vi "Options GFV.vi"(2 "Anything":variant, 5 "error in (no error)":errorcluster, 6 "Action(Get Settings)":T20=enum."Get Settings", 7 "Setting ID":T19=enum."P 2") -> (14 "Update index":i32, 16 "Options":T1={"P 1 (App)"={"Result files"=path "", "PCP Interface"="", "Tractor/Stroker Interface"="", "Tractor Interface"="", "Modem Status Interface"="", "Audible Alarm"=FALSE, "Force alarm on Technical"=FALSE, "Force alarm on HH"=FALSE, "Force alarm on LL"=FALSE, "Force alarm on H"=FALSE, "Force alarm on L"=FALSE}, "P 2"={"Solenoid & Relay latching time"=0, "Tractor relay 1"=0.3, "Tractor relay 2"=0.2, "Tractor Solenoid limit"=0.2}, "P 3"={"Min resistance"=0.0, "Max resistance"=0.0, "Head voltage range"=enum."0 - 350V", "Max voltage jump"=40.0, "Maximum resistance change"=40.0, "Start Telemetry Voltage"=35.0, "Start Telemetry Timeout"=160.0, "Start Motor Voltage"=1.0, "Stop Motor Voltage"=1.0, "Pass Mode Warning Voltage"=1.0, "Relay Switch Voltage"=160.0, "Relay Status Loss Voltage"=0.0, "Samples to average"=1, "PSU type DO NOT USE"=enum."Magna 8.3A", "Magna OVP"=1.0, "Magna Current Limit"=160.0}, "P 4"={"Solenoid & Relay latching time"=40, "Stroker relay 1"=1.0, "Stroker Relay 2"=40.0, "Stroker Solenoid limit"=0.0, "Force det."=enum."Stroke in = node 1", "Stroke force lim."=0.0, "Anchor Enabled Pressure"=0.05, "Tacometer puls"=0.3, "Default anchor behavior"=enum."Do nothing", "Default stroker behavior"=enum."Do nothing", "Default stroker force limit (tonne)"=0.0, "Slips Size"=enum."338 MRS"}, "P 5"={"Solenoid & Relay latching time"=0, "Driller relay 1"=0.3, "Driller Relay 2"=0.2, "Driller  Solenoid limit"=0.2}, "P 6 (Err)"={"Error and event files"=path ""}, "P 7 (Expert)"={"Show Debug"=FALSE, "Log debug messages"=FALSE, "Additional debug messages"=FALSE, "Start Beagle with Simulator data"=FALSE, "Workshop mode"=FALSE, "Modem baud"=38400, "enumCANCOM"=FALSE, "Modem sim"={"Modem dealay sim"=FALSE, "Sim baud Tx"=1200, "Bit Error fraction Tx"=0.0, "Sim baud Rx"=1200, "Bit Error fraction Rx"=0.0}, "Telemetry Timeout Disable"=20, "Buffer size"=20, "Upd regular data"=FALSE, "Cable comp"={"VMOD1 Voltage(V)"=1.0, "VMOD2 Voltage(V)"=8.0}}, "P 8 (Depth)"={"Winch Spool Circumference"=100.0, "Winch Pulses per Revolution"=160.0, "Current Depth"=100.0}, "C 1"={"Depth Updated"=FALSE, "Depth Offset"=0.0}, "C 2"={"Placeholder"=FALSE}} {"P 8 (Depth)"."Current Depth" format="%#.7f"; "P 8 (Depth)"."Winch Pulses per Revolution" min=1.0 max=100000.0 step=1.0 format="%#.0f"; "P 8 (Depth)"."Winch Spool Circumference" min=0.0 max=200.0 format="%#.7f"; "C 1"."Depth Offset" format="%#.7f"; "P 2"."Tractor Solenoid limit" format="%.2f"; "P 2"."Tractor relay 2" format="%.2f"; "P 2"."Tractor relay 1" format="%.2f"; "P 3"."Relay Status Loss Voltage" min=0.0 max=500.0 format="%#.0f"; "P 3"."Relay Switch Voltage" min=5.0 max=500.0 format="%#.0f"; "P 3"."Magna Current Limit" min=0.0 max=20.0 format="%.1f"; "P 3"."Magna OVP" min=0.0 max=1500.0 format="%#.0f"; "P 3"."Pass Mode Warning Voltage" min=5.0 max=500.0 format="%#.0f"; "P 3"."Stop Motor Voltage" min=5.0 max=500.0 format="%#.0f"; "P 3"."Start Telemetry Timeout" min=0.0 max=500.0 format="%#.0f"; "P 3"."Samples to average" min=1 max=10; "P 3"."Start Motor Voltage" min=5.0 max=500.0 format="%#.0f"; "P 3"."Start Telemetry Voltage" min=5.0 max=500.0 format="%#.0f"; "P 3"."Maximum resistance change" min=1.0 max=100.0 format="%#.0f"; "P 3"."Max voltage jump" min=5.0 max=500.0 format="%#.0f"; "P 3"."Max resistance" min=30.0 max=500.0 format="%#.0f"; "P 3"."Min resistance" min=0.0 max=500.0 format="%#.0f"; "P 4"."Default stroker force limit (tonne)" format="%.2f"; "P 4"."Stroker Relay 2" format="%.2f"; "P 4"."Stroker relay 1" format="%.2f"; "P 4"."Tacometer puls" format="%.2f"; "P 4"."Anchor Enabled Pressure" format="%.2f"; "P 4"."Stroke force lim." format="%.2f"; "P 4"."Stroker Solenoid limit" format="%.2f"; "P 5"."Driller  Solenoid limit" format="%.2f"; "P 5"."Driller Relay 2" format="%.2f"; "P 5"."Driller relay 1" format="%.2f"; "P 7 (Expert)"."Cable comp"."VMOD2 Voltage(V)" format="%.1f"; "P 7 (Expert)"."Cable comp"."VMOD1 Voltage(V)" format="%.1f"; "P 7 (Expert)"."Telemetry Timeout Disable" min=2 max=20 step=2; "P 7 (Expert)"."Modem baud" items=["38400 (Normal use)"=38400, "9600 (Development)"=9600]; "P 7 (Expert)"."Modem sim"."Bit Error fraction Rx" format="%.9f"; "P 7 (Expert)"."Modem sim"."Sim baud Rx" items=["9600"=9600, "4800"=4800, "2400"=2400, "1200"=1200, "1000"=1000, "800"=800, "600"=600, "400"=400, "200"=200]; "P 7 (Expert)"."Modem sim"."Bit Error fraction Tx" format="%.9f"; "P 7 (Expert)"."Modem sim"."Sim baud Tx" items=["9600"=9600, "4800"=4800, "2400"=2400, "1200"=1200, "1000"=1000, "800"=800, "600"=600, "400"=400, "200"=200]; "P 7 (Expert)"."Buffer size" min=86400 max=1209600}, 19 "error out":errorcluster)   [LabVIEW 2011]
uses:
  Action GFV Settings.ctl
  Options PageID.ctl
  Options  All pages and custom.ctl
  Options Page 1 (App).ctl
  Options Page 2.ctl
  Options Page 3.ctl
  PCP interface/PCP type List.ctl
  PCP interface/PSU Type.ctl
  Options Page 4.ctl
  Tool/Stroke force selector.ctl
  Tool/Default anchor behavior.ctl
  Tool/Default stroker behavior.ctl
  GUI/Controls/Slips Type Radio.ctl
  Options Page 5.ctl
  Options Page 6 (Err).ctl
  Options Page 7 (Expert).ctl
  GUI/Options/Modem simulation setup.ctl
  Options Page 8 (Depth).ctl
  Options Custom 1.ctl
  Options Custom 2.ctl
  <vilib>/Utility/sysdir.llb/System Directory Type.ctl
  <vilib>/Utility/VariantDataType/GetNumericInfo.vi
  emi Lib/Basic/0 - General/App/Version/Private/_emi_Version Holder.vi
  emi Lib/System 01/0 - General/Debug/Private/_emi_GFV Debug Disp.vi
  emi Lib/System 01/0 - General/Debug/Private/_emi_GFV Debug Log.vi
  emi Lib/System 01/0 - General/Debug/Private/_emi_GFV Debug Aditional.vi
  <vilib>/Utility/libraryn.llb/Check if File or Folder Exists.vi
panel:
  # "m"
  # "Pulses"
  # "Not meant to be directly displayed"
  # "Not meant to be directly displayed"
  # "ms"
  # "When both relays are used in \nthe same operation, the lowest\nlimit is used for both."
  # "A"
  # "A"
  # "A"
  # "Ohm"
  # "Ohm"
  # "V"
  # "Ohm"
  # "V"
  # "s"
  # "V"
  # "V"
  # "V"
  # "V"
  # "V"
  # "ms"
  # "When both relays are used in \nthe same operation, the lowest\nlimit is used for both."
  # "A"
  # "A"
  # "A"
  # "Bar"
  # "ms"
  # "When both relays are used in \nthe same operation, the lowest\nlimit is used for both."
  # "A"
  # "A"
  # "A"
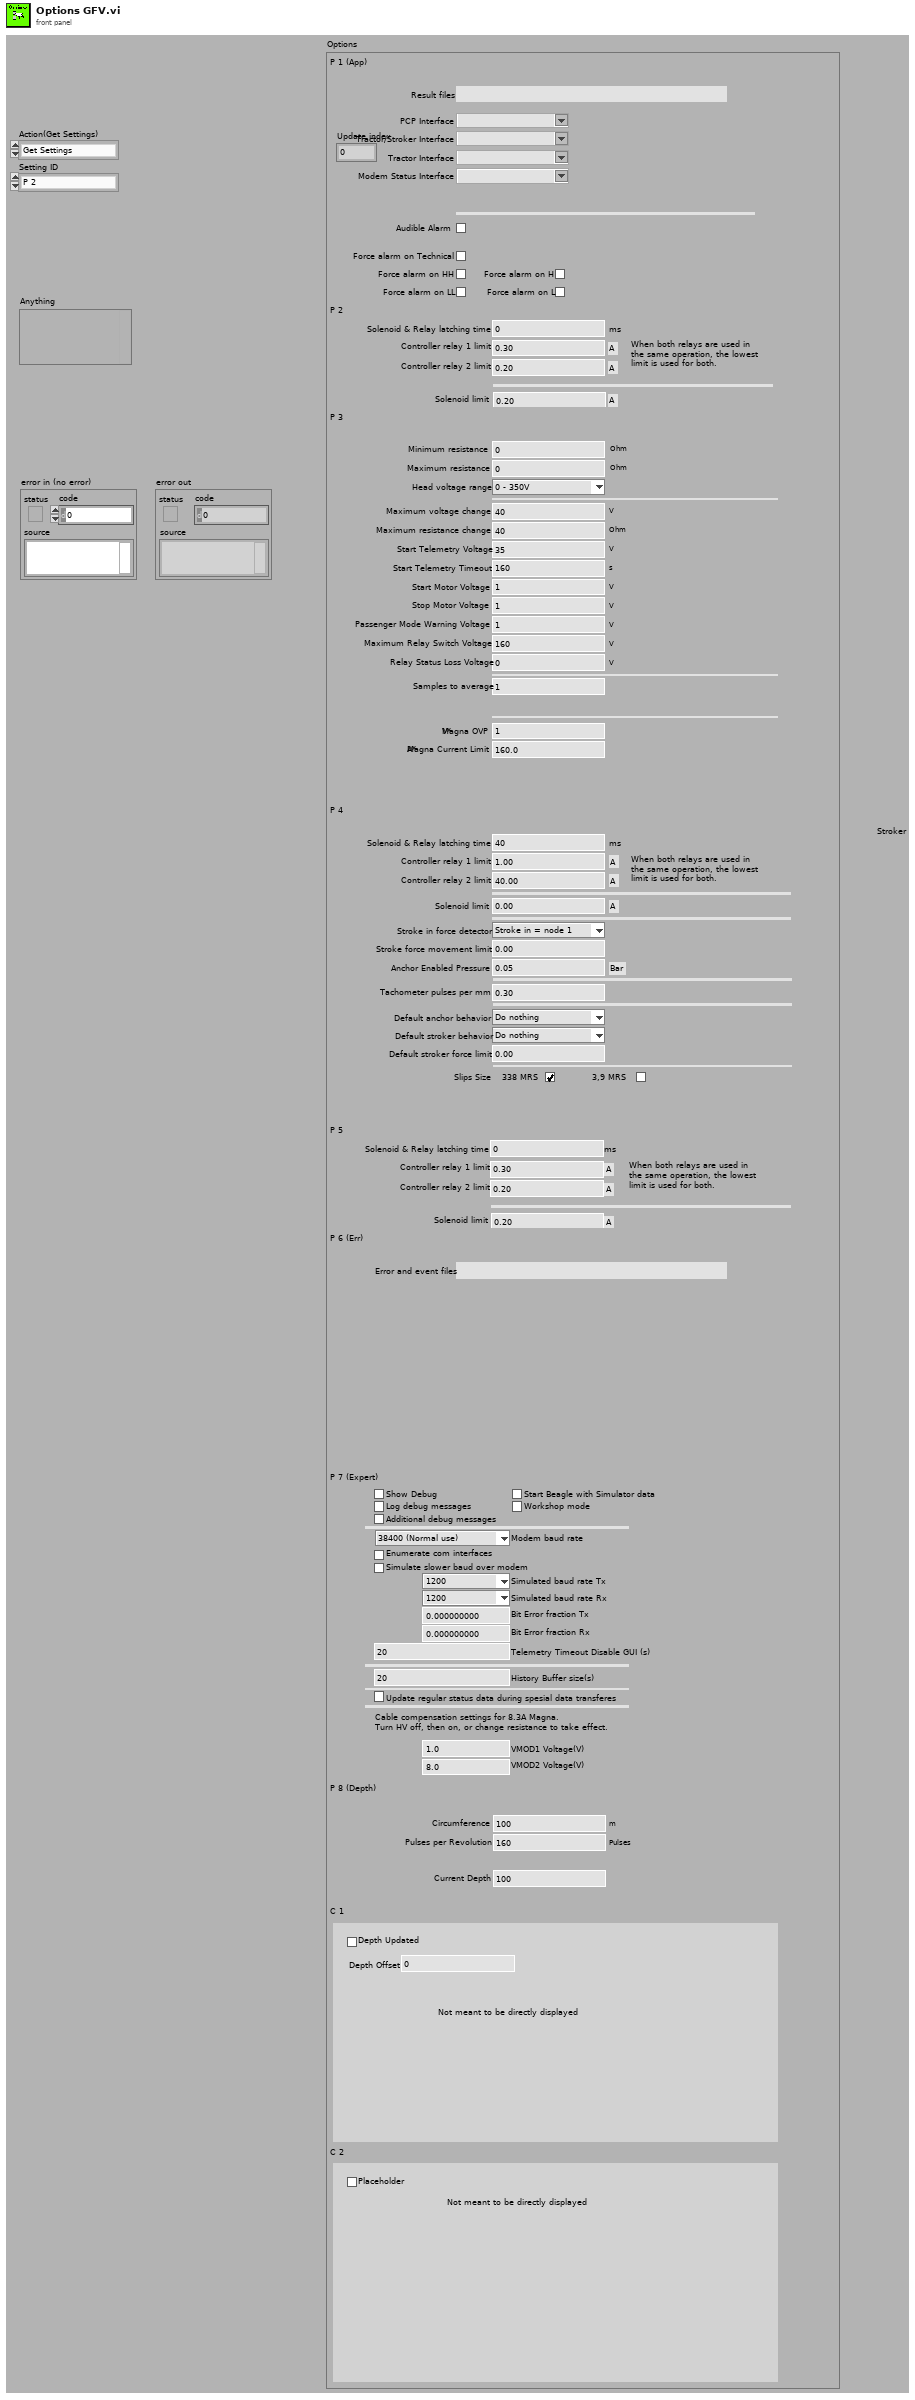
[diagram p1: front panel]
types:
  T1 = typedef "Options  All pages and custom.ctl" = cluster{"P 1 (App)":T2, "P 2":T3, "P 3":T4, "P 4":T7, "P 5":T12, "P 6 (Err)":T13, "P 7 (Expert)":T14, "P 8 (Depth)":T16, "C 1":T17, "C 2":T18}
  T2 = typedef "Options Page 1 (App).ctl" = cluster{"Result files":path, "PCP Interface":string, "Tractor/Stroker Interface":string, "Tractor Interface":string, "Modem Status Interface":string, "Audible Alarm":bool, "Force alarm on Technical":bool, "Force alarm on HH":bool, "Force alarm on LL":bool, "Force alarm on H":bool, "Force alarm on L":bool}
  T3 = typedef "Options Page 2.ctl" = cluster{"Solenoid & Relay latching time":u16, "Tractor relay 1":dbl, "Tractor relay 2":dbl, "Tractor Solenoid limit":dbl}
  T4 = typedef "Options Page 3.ctl" = cluster{"Min resistance":dbl, "Max resistance":dbl, "Head voltage range":T5, "Max voltage jump":dbl, "Maximum resistance change":dbl, "Start Telemetry Voltage":dbl, "Start Telemetry Timeout":dbl, "Start Motor Voltage":dbl, "Stop Motor Voltage":dbl, "Pass Mode Warning Voltage":dbl, "Relay Switch Voltage":dbl, "Relay Status Loss Voltage":dbl, "Samples to average":i32, "PSU type DO NOT USE":T6, "Magna OVP":dbl, "Magna Current Limit":dbl}
  T5 = typedef "PCP type List.ctl" = enum16{"0 - 350V", "0 - 450V", "0 - 600V"}
  T6 = typedef "PSU Type.ctl" = enum16{"Unipower", "Magna 8.3A", "Magna 12A", "None"}
  T7 = typedef "Options Page 4.ctl" = cluster{"Solenoid & Relay latching time":u16, "Stroker relay 1":dbl, "Stroker Relay 2":dbl, "Stroker Solenoid limit":dbl, "Force det.":T8, "Stroke force lim.":dbl, "Anchor Enabled Pressure":dbl, "Tacometer puls":dbl, "Default anchor behavior":T9, "Default stroker behavior":T10, "Default stroker force limit (tonne)":dbl, "Slips Size":T11}
  T8 = typedef "Stroke force selector.ctl" = enum16{"Stroke in = node 1", "Strok out = node 1"}
  T9 = typedef "Default anchor behavior.ctl" = enum16{"Do nothing", "Set Anchor", "Release Anchor"}
  T10 = typedef "Default stroker behavior.ctl" = enum16{"Do nothing", "Stop", "Go Out", "Go In"}
  T11 = typedef "Slips Type Radio.ctl" = enum32{"No Selection", "338 MRS", "3,9 MRS"}
  T12 = typedef "Options Page 5.ctl" = cluster{"Solenoid & Relay latching time":u16, "Driller relay 1":dbl, "Driller Relay 2":dbl, "Driller  Solenoid limit":dbl}
  T13 = typedef "Options Page 6 (Err).ctl" = cluster{"Error and event files":path}
  T14 = typedef "Options Page 7 (Expert).ctl" = cluster{"Show Debug":bool, "Log debug messages":bool, "Additional debug messages":bool, "Start Beagle with Simulator data":bool, "Workshop mode":bool, "Modem baud":u16, "enumCANCOM":bool, "Modem sim":T15, "Telemetry Timeout Disable":i32, "Buffer size":i32, "Upd regular data":bool, "Cable comp":cluster{"VMOD1 Voltage(V)":dbl, "VMOD2 Voltage(V)":dbl}}
  T15 = typedef "Modem simulation setup.ctl" = cluster{"Modem dealay sim":bool, "Sim baud Tx":u16, "Bit Error fraction Tx":dbl, "Sim baud Rx":u16, "Bit Error fraction Rx":dbl}
  T16 = typedef "Options Page 8 (Depth).ctl" = cluster{"Winch Spool Circumference":dbl, "Winch Pulses per Revolution":dbl, "Current Depth":dbl}
  T17 = typedef "Options Custom 1.ctl" = cluster{"Depth Updated":bool, "Depth Offset":dbl}
  T18 = typedef "Options Custom 2.ctl" = cluster{"Placeholder":bool}
  T19 = typedef "Options PageID.ctl" = enum16{"P 1 (App)", "P 2", "P 3", "P 4", "P 5", "P 6 (Err)", "P 7 (Expert)", "P 8", "C 1", "C 2"}
  T20 = typedef "Action GFV Settings.ctl" = enum16{"Init", "Get From INI", "Put In INI", "Get Settings", "Get Update Index", "Set Setting"}
  T21 = enum16{"Set Changed", "Changed?", "Init(numb in Prev..)"}
  T22 = typedef "System Directory Type.ctl" = i32
  T23 = typedef "emi_Version Info.ctl" = cluster{"Name":string, "Major":i16, "Minor":i16, "Fix":i16, "Build":i32, "Type":enum16{"Alfa", "Beta", "Stable"}, "Dev":bool, "Version Name":string, "Date":timestamp}
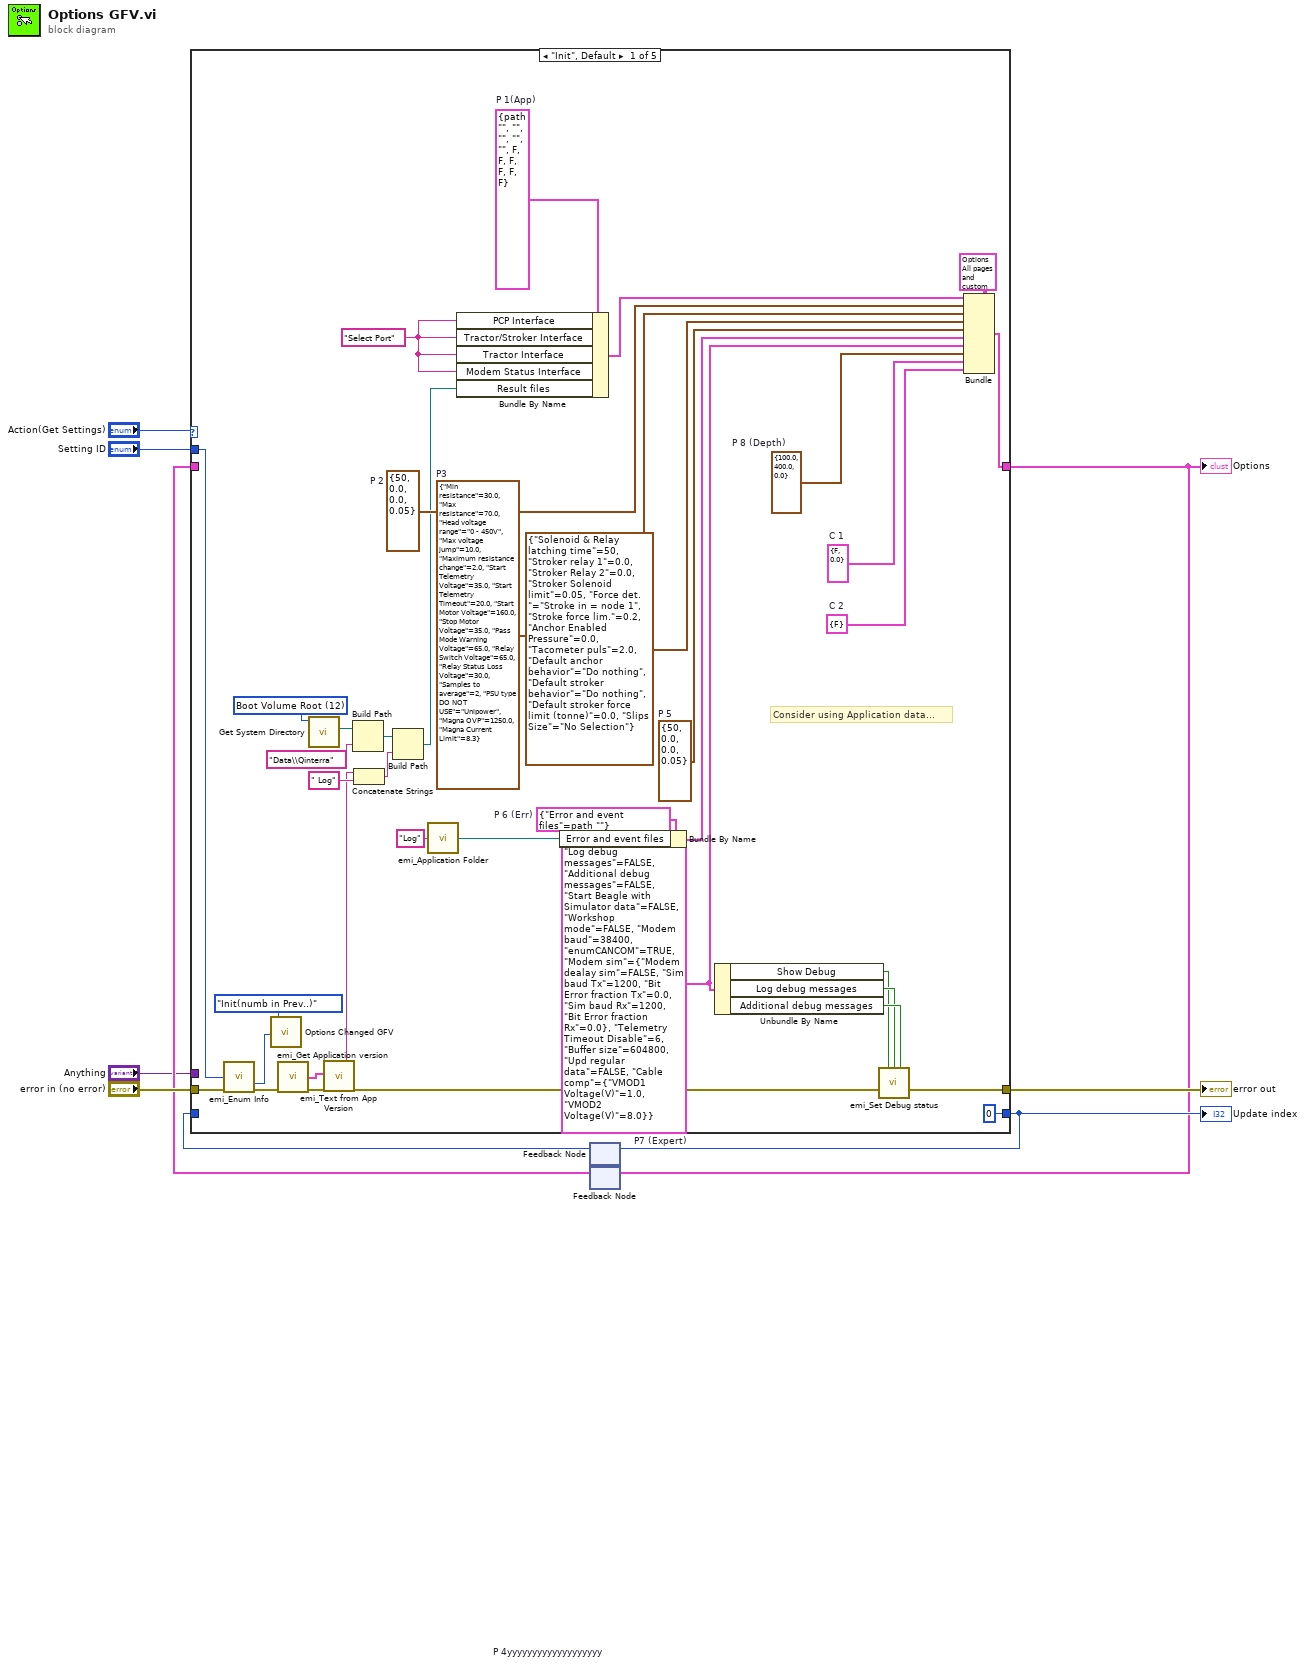
[diagram p0: block diagram]
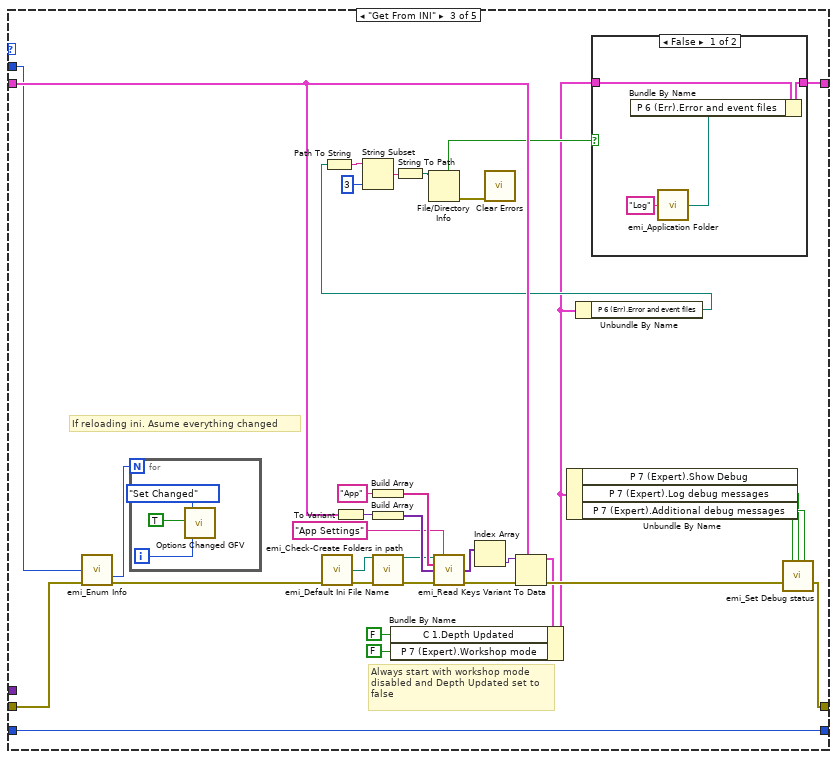
[diagram p3: hidden frame]
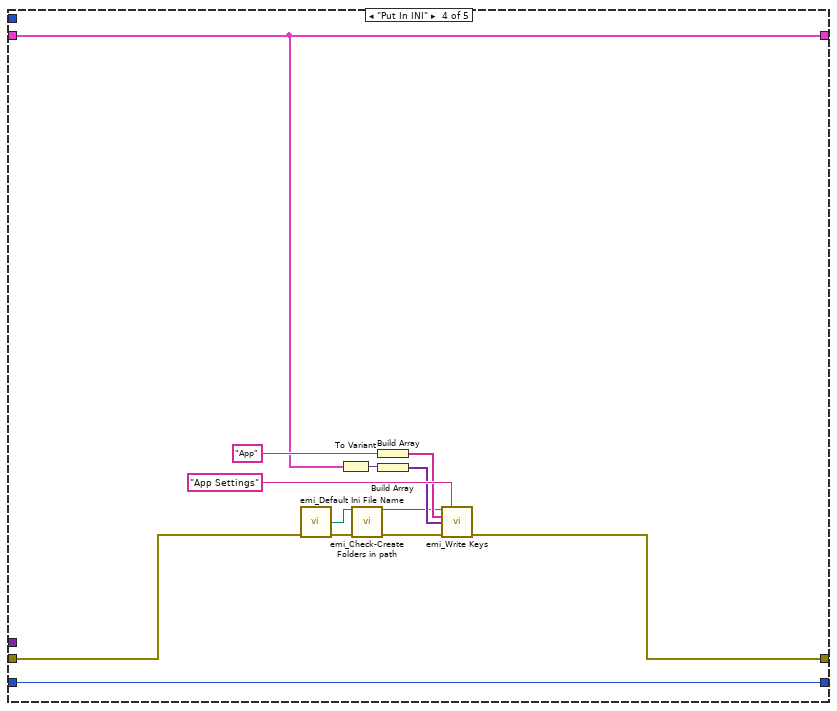
[diagram p5: hidden frame]
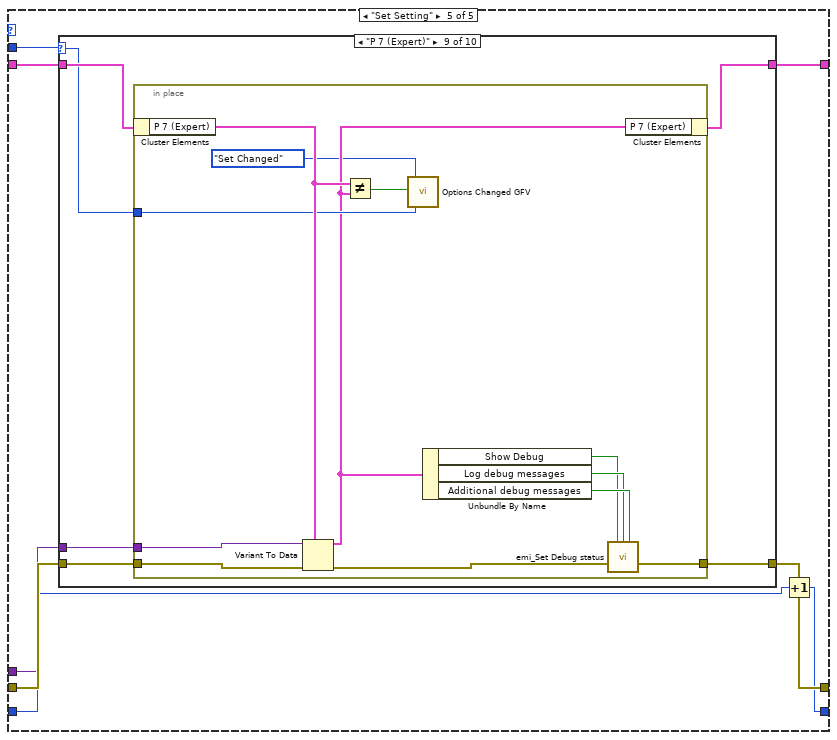
[diagram p6: hidden frame]
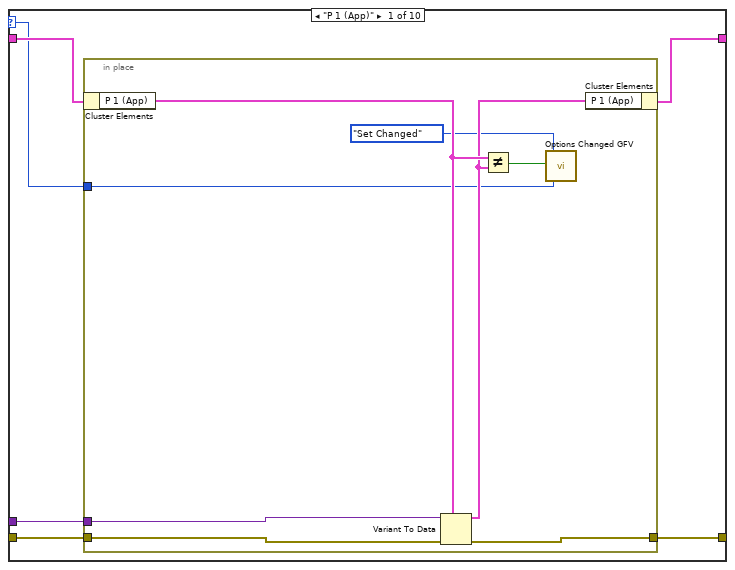
[diagram p7: hidden frame]
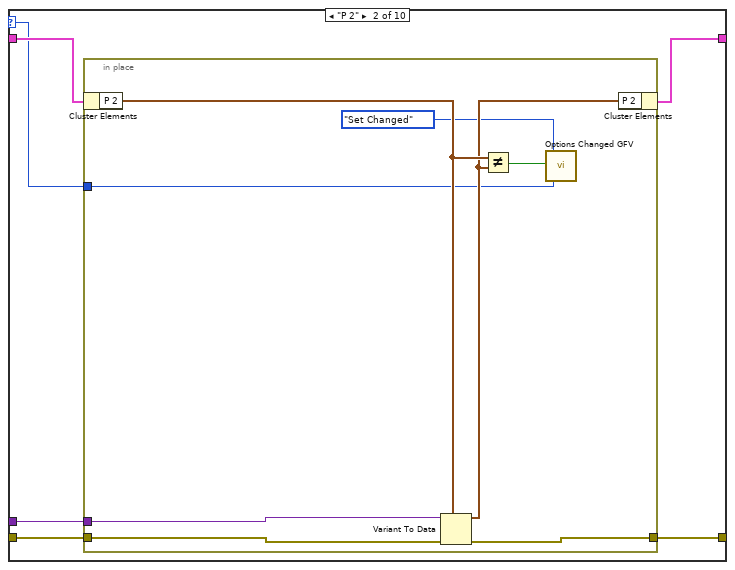
[diagram p8: hidden frame]
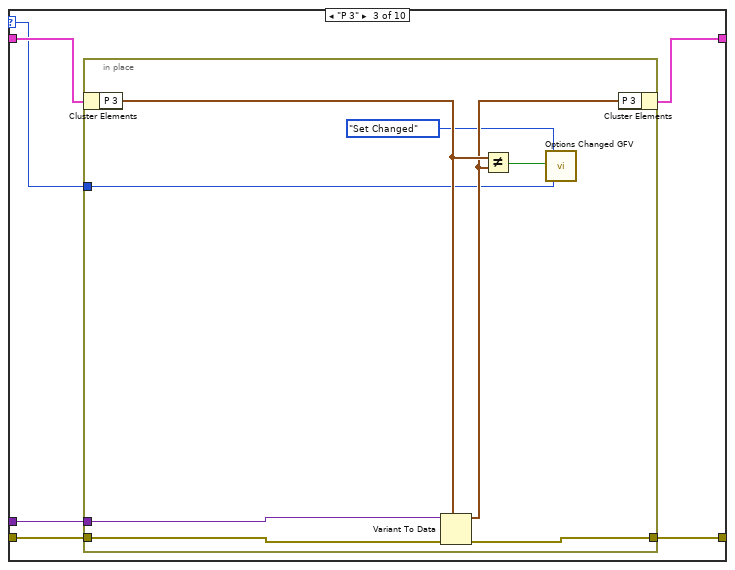
[diagram p9: hidden frame]
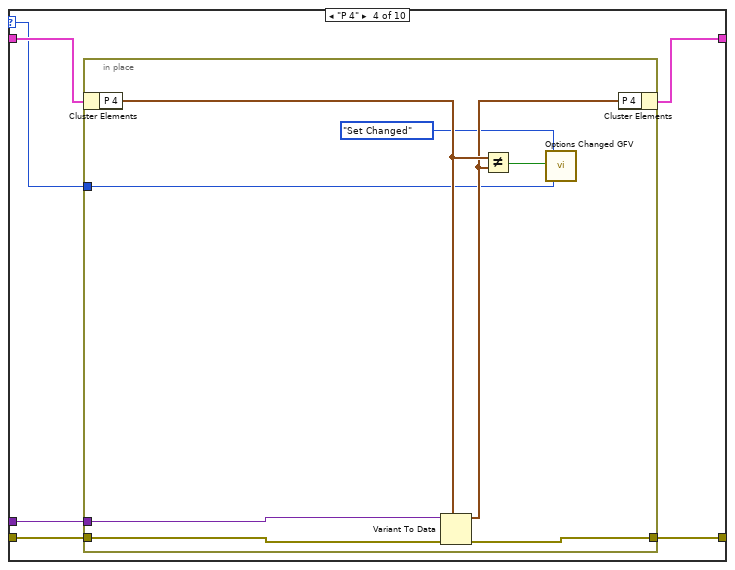
[diagram p10: hidden frame]
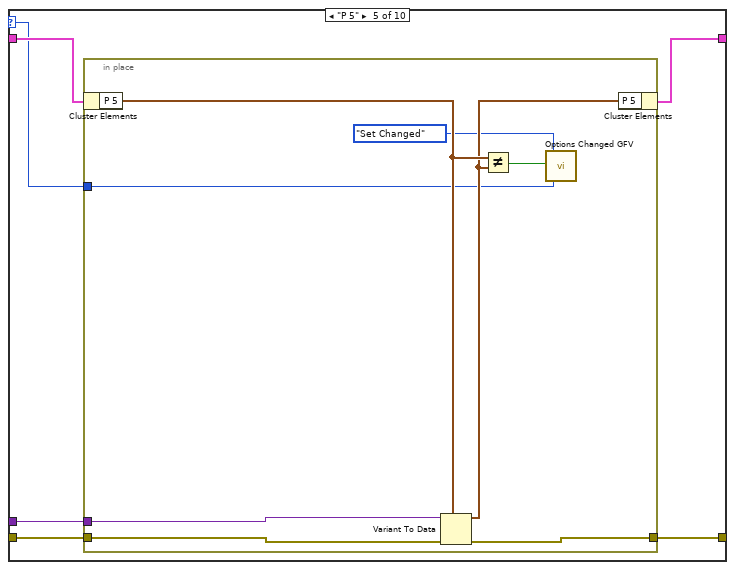
[diagram p11: hidden frame]
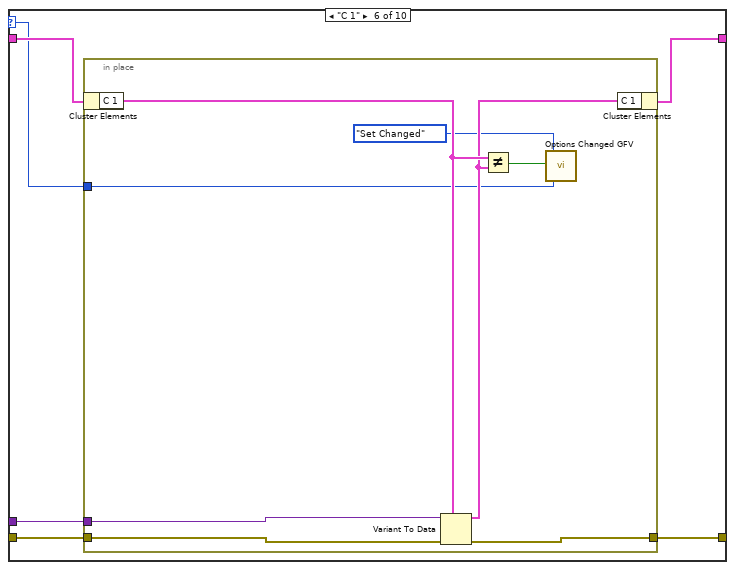
[diagram p12: hidden frame]
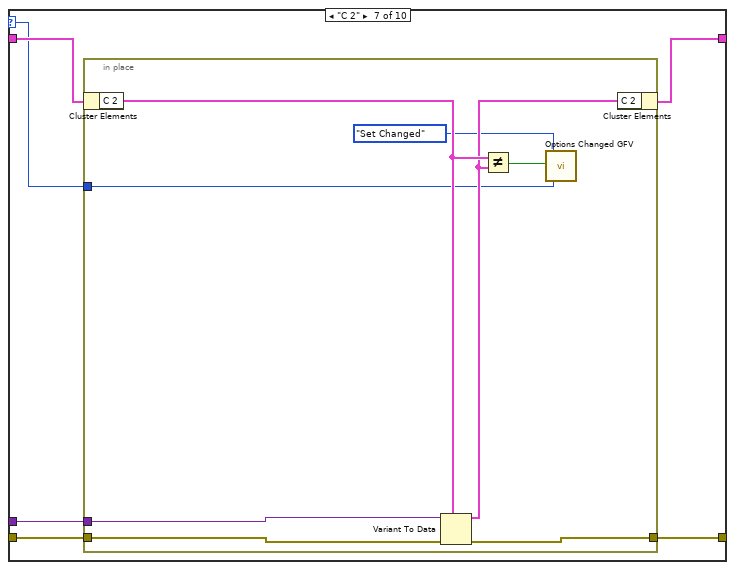
[diagram p13: hidden frame]
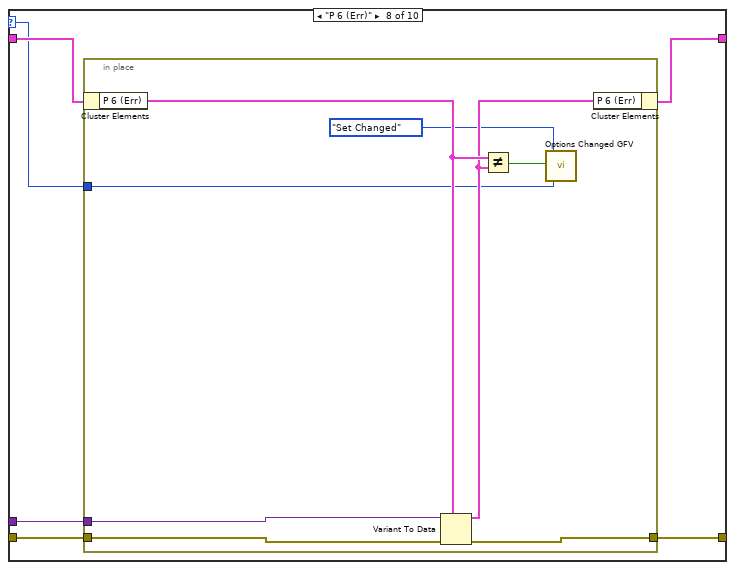
[diagram p14: hidden frame]
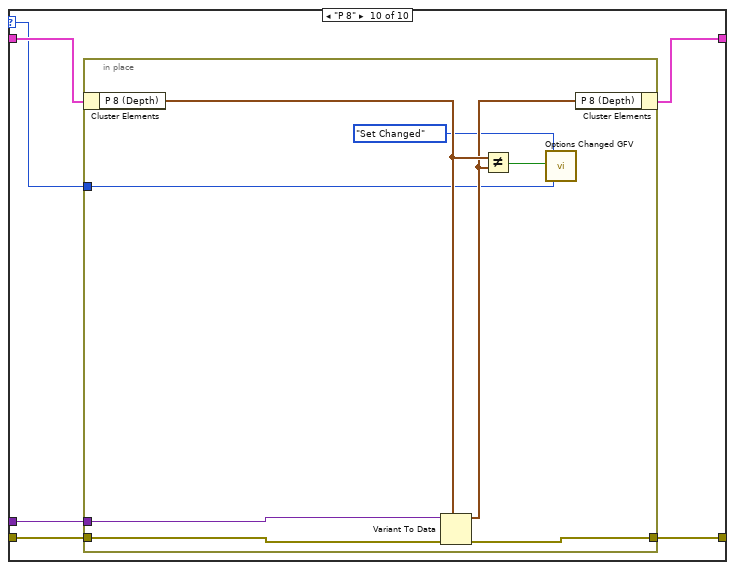
[diagram p15: hidden frame]
diagram:
  n1 = feedback #1() -> (w2:i32)  [unwired: 1 in]
  n2 = feedback #2() -> (w5:T1)  [unwired: 1 in]
  n3 = case shown="\"Init\", Default" "Action(Get Settings)" {
    tunnel: "Setting ID" -> [w31 _ w63 _ w113]
    tunnel: "error in (no error)" -> [w32 w50 w66 w97 w112]
    tunnel: [w36 w50 w67 w100 w111] -> w6
    tunnel: [w46 w49 w55 w104 w109] -> w1
    tunnel: w5 -> [_ w49 w77 w104 w114]
    tunnel: "Anything" -> [_ _ _ _ w110]
    tunnel: [0 w48 w74 w99 w107] -> w3
    tunnel: w2 -> [_ w48 w74 w99 w108]
    frame "Init", Default {
      w10 = T16 {"Winch Spool Circumference"=100.0, "Winch Pulses per Revolution"=400.0, "Current Depth"=0.0}  # P 8 (Depth)
      w14 = "Select Port" ("Modem Interface")
      w16 = T22 12 items=["User Home"=0, "User Desktop"=1, "User Documents"=2, "User Application Data"=3, "User Preferences"=4, "User Temporary"=5, "Public Documents"=6, "Public Application Data"=7, "Public Preferences"=8, "Public Cache"=13, "System Core Libraries"=9, "System Installed Libraries"=10, "Application Files"=11, "Boot Volume Root"=12] ("system directory type")
      w12 = T18 {"Placeholder"=FALSE}  # C 2
      w11 = T17 {"Depth Updated"=FALSE, "Depth Offset"=0.0}  # C 1
      w41 = T7 {"Solenoid & Relay latching time"=50, "Stroker relay 1"=0.0, "Stroker Relay 2"=0.0, "Stroker Solenoid limit"=0.05, "Force det."=enum."Stroke in = node 1", "Stroke force lim."=0.2, "Anchor Enabled Pressure"=0.0, "Tacometer puls"=2.0, "Default anchor behavior"=enum."Do nothing", "Default stroker behavior"=enum."Do nothing", "Default stroker force limit (tonne)"=0.0, "Slips Size"=enum."No Selection"}  # P 4yyyyyyyyyyyyyyyyyyy
      w40 = T12 {"Solenoid & Relay latching time"=50, "Driller relay 1"=0.0, "Driller Relay 2"=0.0, "Driller  Solenoid limit"=0.05}  # P 5
      w42 = T4 {"Min resistance"=30.0, "Max resistance"=70.0, "Head voltage range"=enum."0 - 450V", "Max voltage jump"=10.0, "Maximum resistance change"=2.0, "Start Telemetry Voltage"=35.0, "Start Telemetry Timeout"=20.0, "Start Motor Voltage"=160.0, "Stop Motor Voltage"=35.0, "Pass Mode Warning Voltage"=65.0, "Relay Switch Voltage"=65.0, "Relay Status Loss Voltage"=30.0, "Samples to average"=2, "PSU type DO NOT USE"=enum."Unipower", "Magna OVP"=1250.0, "Magna Current Limit"=8.3}  # P3
      w43 = T3 {"Solenoid & Relay latching time"=50, "Tractor relay 1"=0.0, "Tractor relay 2"=0.0, "Tractor Solenoid limit"=0.05}  # P 2
      w39 = T14 {"Show Debug"=FALSE, "Log debug messages"=FALSE, "Additional debug messages"=FALSE, "Start Beagle with Simulator data"=FALSE, "Workshop mode"=FALSE, "Modem baud"=38400, "enumCANCOM"=TRUE, "Modem sim"={"Modem dealay sim"=FALSE, "Sim baud Tx"=1200, "Bit Error fraction Tx"=0.0, "Sim baud Rx"=1200, "Bit Error fraction Rx"=0.0}, "Telemetry Timeout Disable"=6, "Buffer size"=604800, "Upd regular data"=FALSE, "Cable comp"={"VMOD1 Voltage(V)"=1.0, "VMOD2 Voltage(V)"=8.0}}  # P7 (Expert)
      w27 = T2 {"Result files"=path "", "PCP Interface"="", "Tractor/Stroker Interface"="", "Tractor Interface"="", "Modem Status Interface"="", "Audible Alarm"=FALSE, "Force alarm on Technical"=FALSE, "Force alarm on HH"=FALSE, "Force alarm on LL"=FALSE, "Force alarm on H"=FALSE, "Force alarm on L"=FALSE}  # P 1(App)
      w47 = T13 {"Error and event files"=path ""}  # P 6 (Err)
      # "Consider using Application data..."
      n4 = call "emi_Enum Info.vi"("Enum"=w31, "error in (no error)"=w32) -> ("Numb Elements"=w30:i32, "error out"=w24:errorcluster)  [unwired: 10 in, 2 out]
      n5 = call "Options Changed GFV .vi"("Previous Change No"=w30, "Action(Changed?)"=T21."Init(numb in Prev..)") -> ()  [unwired: 16 in, 2 out]
      n6 = call "emi_Get Application version.vi"("error in (no error)"=w24) -> ("Version Info out"=w25:T23, "error out"=w23:errorcluster)  [unwired: 12 in, 1 out]
      n7 = call <vilib>:"Get System Directory.vi"("system directory type"=w16) -> ("system directory"=w21:path)  [unwired: 10 in]
      n8 = call "emi_Text from App Version.vi"("Version Info"=w25, "error in (no error)"=w23) -> ("Name"=w15:string, "error out"=w22:errorcluster)  [unwired: 8 in, 8 out]
      n9 = Build Path(base path=w21, name or relative path="Data\\Qinterra") -> (appended path=w19:path)
      n10 = Concatenate Strings(w15, " Log" ("string")) -> (w18:string)
      n11 = Build Path(base path=w19, name or relative path=w18) -> (appended path=w13:path)
      n12 = call "emi_Application Folder.vi"("Sub Dir name"="Log") -> ("Dir"=w37:path)  [unwired: 13 in, 1 out]
      n13 = Bundle By Name(cluster=w27, "PCP Interface"=w14, "Tractor/Stroker Interface"=w14, "Tractor Interface"=w14, "Modem Status Interface"=w14, "Result files"=w13) -> (w26:T2)
      n14 = Bundle By Name(cluster=w47, "Error and event files"=w37) -> (w38:T13)
      n15 = Unbundle By Name(w39) -> ("Show Debug"=w33:bool, "Log debug messages"=w34:bool, "Additional debug messages"=w35:bool)
      n16 = call "emi_Set Debug status.vi"("Debug Disp"=w33, "Debug Log"=w34, "Debug Aditional"=w35, "error in (no error)"=w22) -> ("error out"=w36:errorcluster)  [unwired: 11 in]
      n17 = Bundle(cluster=T1 {"P 1 (App)"={"Result files"=path "", "PCP Interface"="", "Tractor/Stroker Interface"="", "Tractor Interface"="", "Modem Status Interface"="", "Audible Alarm"=FALSE, "Force alarm on Technical"=FALSE, "Force alarm on HH"=FALSE, "Force alarm on LL"=FALSE, "Force alarm on H"=FALSE, "Force alarm on L"=FALSE}, "P 2"={"Solenoid & Relay latching time"=0, "Tractor relay 1"=0.0, "Tractor relay 2"=0.0, "Tractor Solenoid limit"=0.0}, "P 3"={"Min resistance"=0.0, "Max resistance"=0.0, "Head voltage range"=enum."0 - 350V", "Max voltage jump"=0.0, "Maximum resistance change"=0.0, "Start Telemetry Voltage"=0.0, "Start Telemetry Timeout"=0.0, "Start Motor Voltage"=0.0, "Stop Motor Voltage"=0.0, "Pass Mode Warning Voltage"=0.0, "Relay Switch Voltage"=0.0, "Relay Status Loss Voltage"=0.0, "Samples to average"=0, "PSU type DO NOT USE"=enum."Unipower", "Magna OVP"=0.0, "Magna Current Limit"=0.0}, "P 4"={"Solenoid & Relay latching time"=0, "Stroker relay 1"=0.0, "Stroker Relay 2"=0.0, "Stroker Solenoid limit"=0.0, "Force det."=enum."Stroke in = node 1", "Stroke force lim."=0.0, "Anchor Enabled Pressure"=0.0, "Tacometer puls"=0.0, "Default anchor behavior"=enum."Do nothing", "Default stroker behavior"=enum."Do nothing", "Default stroker force limit (tonne)"=0.0, "Slips Size"=enum."No Selection"}, "P 5"={"Solenoid & Relay latching time"=0, "Driller relay 1"=0.0, "Driller Relay 2"=0.0, "Driller  Solenoid limit"=0.0}, "P 6 (Err)"={"Error and event files"=path ""}, "P 7 (Expert)"={"Show Debug"=FALSE, "Log debug messages"=FALSE, "Additional debug messages"=FALSE, "Start Beagle with Simulator data"=FALSE, "Workshop mode"=FALSE, "Modem baud"=0, "enumCANCOM"=FALSE, "Modem sim"={"Modem dealay sim"=FALSE, "Sim baud Tx"=0, "Bit Error fraction Tx"=0.0, "Sim baud Rx"=0, "Bit Error fraction Rx"=0.0}, "Telemetry Timeout Disable"=0, "Buffer size"=0, "Upd regular data"=FALSE, "Cable comp"={"VMOD1 Voltage(V)"=0.0, "VMOD2 Voltage(V)"=0.0}}, "P 8 (Depth)"={"Winch Spool Circumference"=0.0, "Winch Pulses per Revolution"=0.0, "Current Depth"=0.0}, "C 1"={"Depth Updated"=FALSE, "Depth Offset"=0.0}, "C 2"={"Placeholder"=FALSE}} ("Options"), "P 1 (App)"=w26, "P 2"=w43, "P 3"=w42, "P 4"=w41, "P 5"=w40, "P 6 (Err)"=w38, "P 7 (Expert)"=w39, "P 8 (Depth)"=w10, "C 1"=w11, "C 2"=w12) -> (w46:T1)
    }
    frame "Get Settings", "Get Update Index" {
      # "Get update index is to se if updated without unpacking cluster"
    }
    frame "Get From INI" {
      # "Always start with workshop mode\ndisabled and Depth Updated set to\nfalse"
      # "If reloading ini. Asume everything changed"
      n18 = call "emi_Enum Info.vi"("Enum"=w63, "error in (no error)"=w66) -> ("Numb Elements"=w65:i32, "error out"=w64:errorcluster)  [unwired: 10 in, 2 out]
      n19 = for {
        N: w65 -> [_]
        i -> [w91]
        n20 = call "Options Changed GFV .vi"("Changed"=TRUE, "Action(Changed?)"=T21."Set Changed", "Setting ID"=w91) -> ()  [unwired: 15 in, 2 out]
      }
      n21 = call "emi_Default Ini File Name.vi"("error in (no error)"=w64) -> ("Path"=w73:path, "error out"=w85:errorcluster)  [unwired: 13 in]
      n22 = To Variant(anything=w77) -> (Variant=w80:variant)
      n23 = Build Array("App" ("Section")) -> (w83:string[])
      n24 = Build Array(w80) -> (w82:variant[])
      n25 = call "emi_Check-Create Folders in path.vi"("Path including file"=w73, "error in (no error)"=w85) -> ("Path out"=w72:path, "error out"=w84:errorcluster)  [unwired: 11 in, 1 out]
      n26 = call "emi_Read Keys.vi"("Ini Path(..app../config.ini)"=w72, "Section"="App Settings", "Key Names"=w83, "Types/Defaults"=w82, "error in (no error)"=w84) -> ("Values"=w76:variant[], "error out"=w78:errorcluster)  [unwired: 8 in, 1 out]
      n27 = Index Array(array=w76) -> (element=w75:variant)  [unwired: 1 in]
      n28 = Variant To Data(error in=w78, type=w77, Variant=w75) -> (data=w54:T1, error out=w68:errorcluster)
      n29 = Bundle By Name(cluster=w54, "C 1.Depth Updated"=FALSE, "P 7 (Expert).Workshop mode"=FALSE) -> (w53:T1)
      n30 = Unbundle By Name(w53) -> ("P 7 (Expert).Show Debug"=w69:bool, "P 7 (Expert).Log debug messages"=w70:bool, "P 7 (Expert).Additional debug messages"=w71:bool)
      n31 = Unbundle By Name(w53) -> ("P 6 (Err).Error and event files"=w57:path)
      n32 = Path To String(path=w57) -> (string=w58:string)
      n33 = String Subset(string=w58, length (rest)=3 ("length (rest)")) -> (substring=w60:string)  [unwired: 1 in]
      n34 = String To Path(string=w60) -> (path=w62:path)
      n35 = File/Directory Info(path=w62) -> (directory=w56:bool, error out=w61:errorcluster)  [unwired: 1 in, 5 out]
      n36 = call <vilib>:"Clear Errors.vi"("error in (no error)"=w61) -> ()  [unwired: 6 in, 1 out]
      n37 = case shown="False" w56 {
        tunnel: w53 -> [w88 w90]
        tunnel: [w87 w90] -> w55
        frame False {
          n38 = call "emi_Application Folder.vi"("Sub Dir name"="Log") -> ("Dir"=w86:path)  [unwired: 13 in, 1 out]
          n39 = Bundle By Name(cluster=w88, "P 6 (Err).Error and event files"=w86) -> (w87:T1)
        }
        frame True {
        }
      }
      n40 = call "emi_Set Debug status.vi"("Debug Disp"=w69, "Debug Log"=w70, "Debug Aditional"=w71, "error in (no error)"=w68) -> ("error out"=w67:errorcluster)  [unwired: 11 in]
    }
    frame "Put In INI" {
      n41 = call "emi_Default Ini File Name.vi"("error in (no error)"=w97) -> ("Path"=w98:path, "error out"=w96:errorcluster)  [unwired: 13 in]
      n42 = To Variant(anything=w104) -> (Variant=w106:variant)
      n43 = call "emi_Check-Create Folders in path.vi"("Path including file"=w98, "error in (no error)"=w96) -> ("Path out"=w95:path, "error out"=w94:errorcluster)  [unwired: 11 in, 1 out]
      n44 = Build Array("App" ("Section")) -> (w102:string[])
      n45 = Build Array(w106) -> (w101:variant[])
      n46 = call "emi_Write Keys.vi"("Ini Path(..app../config.ini)"=w95, "Section"="App Settings", "Key Names"=w102, "Values"=w101, "error in (no error)"=w94) -> ("error out"=w100:errorcluster)  [unwired: 9 in, 1 out]
    }
    frame "Set Setting" {
      n47 = case shown="\"P 7 (Expert)\"" w113 {
        selector: w113 -> [w115 w129 w143 w157 w171 w185 w199 w213 w227 w245]
        tunnel: w114 -> [w120 w134 w148 w162 w176 w190 w204 w218 w232 w250]
        tunnel: w112 -> [w118 w132 w146 w160 w174 w188 w202 w216 w230 w248]
        tunnel: [w116 w130 w144 w158 w172 w186 w200 w214 w228 w246] -> w111
        tunnel: w110 -> [w117 w131 w145 w159 w173 w187 w201 w215 w229 w247]
        tunnel: [w119 w133 w147 w161 w175 w189 w203 w217 w231 w249] -> w109
        frame "P 1 (App)" {
          n48 = in-place {
            in-place-border: w118 -> [w128]
            in-place-border: w117 -> [w127]
            in-place-border: [w122] -> w116
            in-place-border: w115 -> [w123]
            n49 = in-place-cluster #3(w120) -> ("P 1 (App)"=w126:T2)
            n50 = Variant To Data(error in=w128, type=w126, Variant=w127) -> (data=w125:T2, error out=w122:errorcluster)
            n51 = Not Equal?(x=w126, y=w125) -> (x != y?=w124:bool)
            n52 = call "Options Changed GFV .vi"("Changed"=w124, "Action(Changed?)"=T21."Set Changed", "Setting ID"=w123) -> ()  [unwired: 15 in, 2 out]
            n53 = in-place-cluster #3("P 1 (App)"=w125) -> (w119:T1)
          }
        }
        frame "P 2" {
          n54 = in-place {
            in-place-border: w132 -> [w142]
            in-place-border: w131 -> [w141]
            in-place-border: [w136] -> w130
            in-place-border: w129 -> [w137]
            n55 = in-place-cluster #4(w134) -> ("P 2"=w140:T3)
            n56 = Variant To Data(error in=w142, type=w140, Variant=w141) -> (data=w139:T3, error out=w136:errorcluster)
            n57 = Not Equal?(x=w140, y=w139) -> (x != y?=w138:bool)
            n58 = call "Options Changed GFV .vi"("Changed"=w138, "Action(Changed?)"=T21."Set Changed", "Setting ID"=w137) -> ()  [unwired: 15 in, 2 out]
            n59 = in-place-cluster #4("P 2"=w139) -> (w133:T1)
          }
        }
        frame "P 3" {
          n60 = in-place {
            in-place-border: w146 -> [w156]
            in-place-border: w145 -> [w155]
            in-place-border: [w150] -> w144
            in-place-border: w143 -> [w151]
            n61 = in-place-cluster #5(w148) -> ("P 3"=w154:T4)
            n62 = Variant To Data(error in=w156, type=w154, Variant=w155) -> (data=w153:T4, error out=w150:errorcluster)
            n63 = Not Equal?(x=w154, y=w153) -> (x != y?=w152:bool)
            n64 = call "Options Changed GFV .vi"("Changed"=w152, "Action(Changed?)"=T21."Set Changed", "Setting ID"=w151) -> ()  [unwired: 15 in, 2 out]
            n65 = in-place-cluster #5("P 3"=w153) -> (w147:T1)
          }
        }
        frame "P 4" {
          n66 = in-place {
            in-place-border: w160 -> [w170]
            in-place-border: w159 -> [w169]
            in-place-border: [w164] -> w158
            in-place-border: w157 -> [w165]
            n67 = in-place-cluster #6(w162) -> ("P 4"=w168:T7)
            n68 = Variant To Data(error in=w170, type=w168, Variant=w169) -> (data=w167:T7, error out=w164:errorcluster)
            n69 = Not Equal?(x=w168, y=w167) -> (x != y?=w166:bool)
            n70 = call "Options Changed GFV .vi"("Changed"=w166, "Action(Changed?)"=T21."Set Changed", "Setting ID"=w165) -> ()  [unwired: 15 in, 2 out]
            n71 = in-place-cluster #6("P 4"=w167) -> (w161:T1)
          }
        }
        frame "P 5" {
          n72 = in-place {
            in-place-border: w174 -> [w184]
            in-place-border: w173 -> [w183]
            in-place-border: [w178] -> w172
            in-place-border: w171 -> [w179]
            n73 = in-place-cluster #7(w176) -> ("P 5"=w182:T12)
            n74 = Variant To Data(error in=w184, type=w182, Variant=w183) -> (data=w181:T12, error out=w178:errorcluster)
            n75 = Not Equal?(x=w182, y=w181) -> (x != y?=w180:bool)
            n76 = call "Options Changed GFV .vi"("Changed"=w180, "Action(Changed?)"=T21."Set Changed", "Setting ID"=w179) -> ()  [unwired: 15 in, 2 out]
            n77 = in-place-cluster #7("P 5"=w181) -> (w175:T1)
          }
        }
        frame "C 1" {
          n78 = in-place {
            in-place-border: w188 -> [w198]
            in-place-border: w187 -> [w197]
            in-place-border: [w192] -> w186
            in-place-border: w185 -> [w193]
            n79 = in-place-cluster #8(w190) -> ("C 1"=w196:T17)
            n80 = Variant To Data(error in=w198, type=w196, Variant=w197) -> (data=w195:T17, error out=w192:errorcluster)
            n81 = Not Equal?(x=w196, y=w195) -> (x != y?=w194:bool)
            n82 = call "Options Changed GFV .vi"("Changed"=w194, "Action(Changed?)"=T21."Set Changed", "Setting ID"=w193) -> ()  [unwired: 15 in, 2 out]
            n83 = in-place-cluster #8("C 1"=w195) -> (w189:T1)
          }
        }
        frame "C 2" {
          n84 = in-place {
            in-place-border: w202 -> [w212]
            in-place-border: w201 -> [w211]
            in-place-border: [w206] -> w200
            in-place-border: w199 -> [w207]
            n85 = in-place-cluster #9(w204) -> ("C 2"=w210:T18)
            n86 = Variant To Data(error in=w212, type=w210, Variant=w211) -> (data=w209:T18, error out=w206:errorcluster)
            n87 = Not Equal?(x=w210, y=w209) -> (x != y?=w208:bool)
            n88 = call "Options Changed GFV .vi"("Changed"=w208, "Action(Changed?)"=T21."Set Changed", "Setting ID"=w207) -> ()  [unwired: 15 in, 2 out]
            n89 = in-place-cluster #9("C 2"=w209) -> (w203:T1)
          }
        }
        frame "P 6 (Err)" {
          n90 = in-place {
            in-place-border: w216 -> [w226]
            in-place-border: w215 -> [w225]
            in-place-border: [w220] -> w214
            in-place-border: w213 -> [w221]
            n91 = in-place-cluster #10(w218) -> ("P 6 (Err)"=w224:T13)
            n92 = Variant To Data(error in=w226, type=w224, Variant=w225) -> (data=w223:T13, error out=w220:errorcluster)
            n93 = Not Equal?(x=w224, y=w223) -> (x != y?=w222:bool)
            n94 = call "Options Changed GFV .vi"("Changed"=w222, "Action(Changed?)"=T21."Set Changed", "Setting ID"=w221) -> ()  [unwired: 15 in, 2 out]
            n95 = in-place-cluster #10("P 6 (Err)"=w223) -> (w217:T1)
          }
        }
        frame "P 7 (Expert)" {
          n96 = in-place {
            in-place-border: w230 -> [w244]
            in-place-border: w229 -> [w243]
            in-place-border: [w235] -> w228
            in-place-border: w227 -> [w240]
            n97 = in-place-cluster #11(w232) -> ("P 7 (Expert)"=w242:T14)
            n98 = Variant To Data(error in=w244, type=w242, Variant=w243) -> (data=w234:T14, error out=w236:errorcluster)
            n99 = Not Equal?(x=w242, y=w234) -> (x != y?=w241:bool)
            n100 = call "Options Changed GFV .vi"("Changed"=w241, "Action(Changed?)"=T21."Set Changed", "Setting ID"=w240) -> ()  [unwired: 15 in, 2 out]
            n101 = Unbundle By Name(w234) -> ("Show Debug"=w237:bool, "Log debug messages"=w238:bool, "Additional debug messages"=w239:bool)
            n102 = call "emi_Set Debug status.vi"("Debug Disp"=w237, "Debug Log"=w238, "Debug Aditional"=w239, "error in (no error)"=w236) -> ("error out"=w235:errorcluster)  [unwired: 11 in]
            n103 = in-place-cluster #11("P 7 (Expert)"=w234) -> (w231:T1)
          }
        }
        frame "P 8" {
          n104 = in-place {
            in-place-border: w248 -> [w258]
            in-place-border: w247 -> [w257]
            in-place-border: [w252] -> w246
            in-place-border: w245 -> [w253]
            n105 = in-place-cluster #12(w250) -> ("P 8 (Depth)"=w256:T16)
            n106 = Variant To Data(error in=w258, type=w256, Variant=w257) -> (data=w255:T16, error out=w252:errorcluster)
            n107 = Not Equal?(x=w256, y=w255) -> (x != y?=w254:bool)
            n108 = call "Options Changed GFV .vi"("Changed"=w254, "Action(Changed?)"=T21."Set Changed", "Setting ID"=w253) -> ()  [unwired: 15 in, 2 out]
            n109 = in-place-cluster #12("P 8 (Depth)"=w255) -> (w249:T1)
          }
        }
      }
      n110 = Increment(x=w108) -> (x+1=w107:i32)
    }
  }
  "error out" <- w6
  "Options" <- w1
  "Update index" <- w3
  n111 = feedback-in #1(w3) -> ()
  n112 = feedback-in #2(w1) -> ()
